vi "Begin.vi"(8 "error in":errorcluster) -> (0 "error out":errorcluster)   [LabVIEW 2018]
doc: "Called before other user functions, this VI is expected to open initial I/O refnums, load in file data, and do all program initialization. Notice that the <B>error out</B> terminal is simply used for data flow. Wiring it to other structures or subVIs ensures that this VI runs first."
uses:
  <vilib>/Rock Robotics/WPI/SafetyOutput/WPI_SafetyOutputConfigMenu.ctl
  <vilib>/Rock Robotics/WPI/DriverStation/WPI_DriverStationRobotMode2.ctl
  <vilib>/Rock Robotics/WPI/Joystick/WPI_JoystickDeviceEnum.ctl
  <vilib>/Rock Robotics/SystemInterfaces/DIO/FPGA_DIOPWMChannel.ctl
  Robot Global Data.vi
  <vilib>/Rock Robotics/Network Tables/NT Write String Array.vi
  <vilib>/Rock Robotics/WPI/RobotDrive/WPI_RobotDriveOpen4MotorWithJaguar.vi
  <vilib>/Rock Robotics/WPI/Solenoid/WPI_SolenoidChannel.ctl
  <vilib>/Rock Robotics/WPI/MotorControl/WPI_MotorControlOpen SPARK.vi
  <vilib>/Rock Robotics/WPI/Solenoid/WPI_SolenoidOpenDouble.vi
  <vilib>/Rock Robotics/WPI/ThirdParty/REV Robotics/SPARK MAX/Typedef/Spark MAX Motor Type.ctl
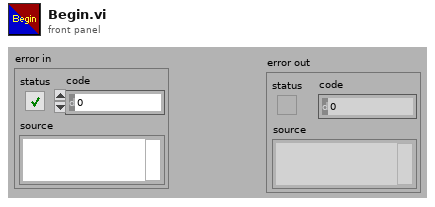
[diagram p1: front panel]
types:
  T1 = typedef "FPGA_DIOPWMChannel.ctl" = enum8{"PWM 0", "PWM 1", "PWM 2", "PWM 3", "PWM 4", "PWM 5", "PWM 6", "PWM 7", "PWM 8", "PWM 9", "PWM MXP 0", "PWM MXP 1", "PWM MXP 2", "PWM MXP 3", "PWM MXP 4", "PWM MXP 5", "PWM MXP 6", "PWM MXP 7", "PWM MXP 8", "PWM MXP 9", "Invalid"}
  T2 = typedef "WPI_JoystickDeviceEnum.ctl" = enum16{"USB 0", "USB 1", "USB 2", "USB 3", "USB 4", "USB 5"}
  T3 = typedef "WPI_DriverStationRobotMode2.ctl" = enum16{"Autonomous Disabled", "Autonomous Enabled", "Teleop Disabled", "Teleop Enabled", "Disconnected", "Finish", "Test Disabled", "Test Enabled", "Emergency Stopped"}
  T4 = typedef "WPI_SafetyOutputConfigMenu.ctl" = enum16{"Enable", "Disable"}
  T5 = typedef "Spark MAX Motor Type.ctl" = enum16{"Brushed", "Brushless"}
  T6 = cluster{"P Gain":dbl, "I Gain":dbl, "D Gain":dbl, "F Gain":dbl, "I Zone":dbl, "Min Output":dbl, "Max Output":dbl}
  T7 = typedef "WPI_SolenoidChannel.ctl" = enum8{"Solenoid 0", "Solenoid 1", "Solenoid 2", "Solenoid 3", "Solenoid 4", "Solenoid 5", "Solenoid 6", "Solenoid 7", "Invalid"}
  T8 = typedef "WPI_MotorControlDeviceRef.ctl" = cluster{"DeviceStatus":errorcluster, "Type":T9, "PWM":cluster{"PWM Channel":T1, "DeadBand":T10}, "CAN":cluster{"Device Number":u8, "SetOutput VI Ref":variant, "GetOutput VI Ref":variant, "Enable VI Ref":variant, "Disable VI Ref":variant, "Data":variant}, "Invert":bool, "DIO PWM":cluster{"PWM \"Enable\" Channel":T1, "DIOChannel":T11, "PWM Rate":dbl}}
  T9 = typedef "WPI_MotorControlType.ctl" = enum16{"PWM", "CAN", "DIO PWM"}
  T10 = typedef "WPI_PWMDeadband.ctl" = cluster{"Name":string, "maxPositivePwm":i32, "minPositivePwm":i32, "centerPwm":i32, "maxNegativePwm":i32, "minNegativePwm":i32, "angularRange":u16}
  T11 = typedef "FPGA_DIOChannel.ctl" = enum8{"DIO 0", "DIO 1", "DIO 2", "DIO 3", "DIO 4", "DIO 5", "DIO 6", "DIO 7", "DIO 8", "DIO 9", "DIO MXP 0", "DIO MXP 1", "DIO MXP 2", "DIO MXP 3", "DIO MXP 4", "DIO MXP 5", "DIO MXP 6", "DIO MXP 7", "DIO MXP 8", "DIO MXP 9", "DIO MXP 10", "DIO MXP 11", "DIO MXP 12", "DIO MXP 13", "DIO MXP 14", "DIO MXP 15", "SPI Port CS1", "SPI Port CS2", "SPI Port CS3", "SPI Port MISO", "SPI Port MOSI", "Invalid"}
  T12 = typedef "WPI_SolenoidDevRef.ctl" = cluster{"DevStatus":errorcluster, "Pneumatics Control Module":u8, "Forward Solenoid Channel":T7, "Reverse Solenoid Channel":T7}
  T13 = typedef "WPI_CompressorDevRef.ctl" = cluster{"DevStatus":errorcluster, "Pneumatics Control Module":u8}
  T14 = typedef "WPI_CameraDevRef.ctl" = cluster{"Camera Address":string, "CameraStatus":errorcluster}
  T15 = typedef "WPI_RobotDriveDevRef.ctl" = cluster{"DevStatus":errorcluster, "Motors[]":T8[], "Square Inputs":bool, "Max Output":dbl}
  T16 = typedef "WPI_JoystickDevRef.ctl" = cluster{"Device":T2}
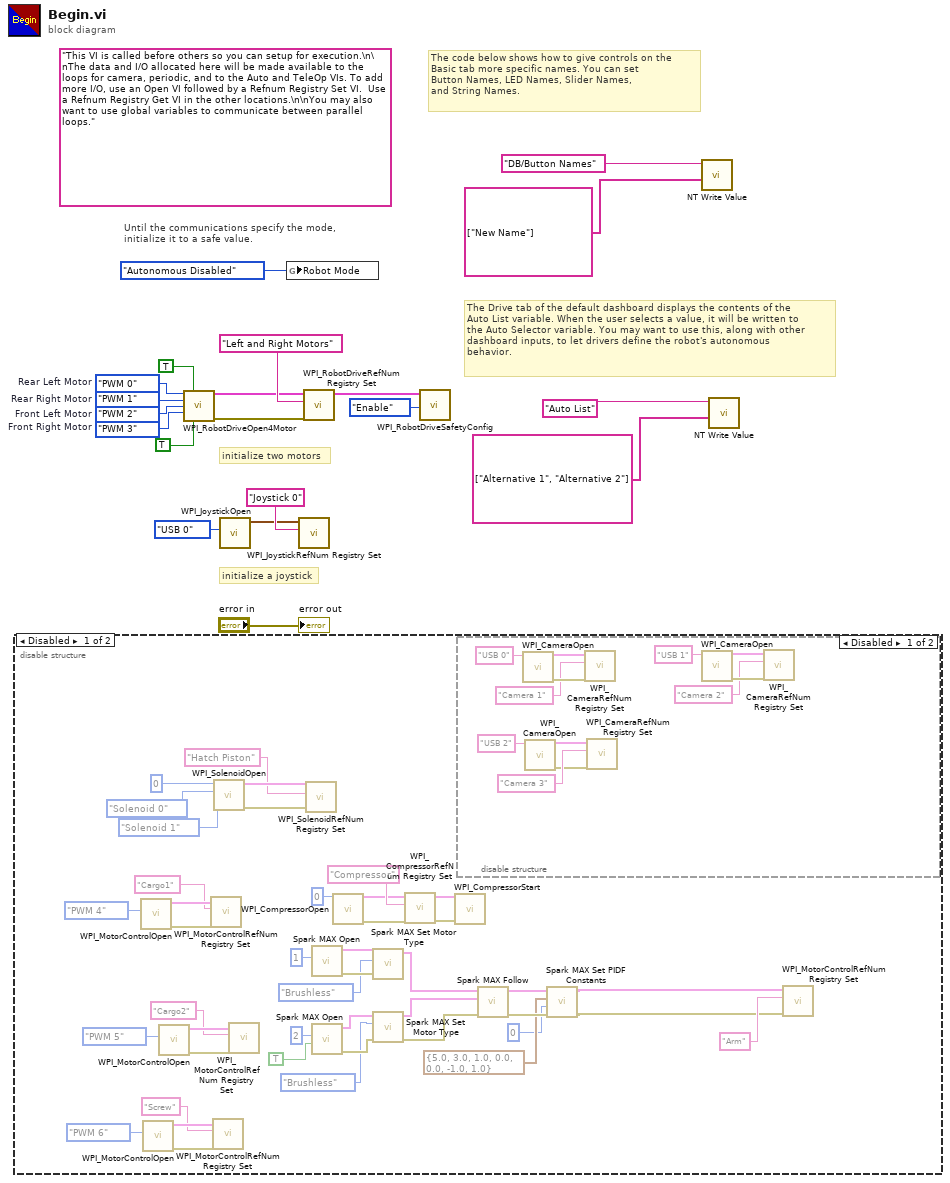
[diagram p0: block diagram]
diagram:
  w3 = FPGA_DIOPWMChannel."PWM 3"  # Front Right Motor
  w4 = FPGA_DIOPWMChannel."PWM 2"  # Front Left Motor
  w5 = FPGA_DIOPWMChannel."PWM 1"  # Rear Right Motor
  w6 = FPGA_DIOPWMChannel."PWM 0"  # Rear Left Motor
  (unwired) "This VI is called before others so you can setup for execution.\n\nThe data and I/O allocated here will be made available to the loops for camera, periodic, and to the Auto and TeleOp VIs. To add more I/O, use an Open VI followed by a Refnum Registry Set VI.  Use a Refnum Registry Get VI in the other locations.\n\nYou may also want to use global variables to communicate between parallel loops."
  # "The Drive tab of the default dashboard displays the contents of the\nAuto List variable. When the user selects a value, it will be written to\nthe Auto Selector variable. You may want to use this, along with other\ndashboard inputs, to let drivers define the robot's autonomous\nbehavior."
  # "The code below shows how to give controls on the\nBasic tab more specific names. You can set\nButton Names, LED Names, Slider Names,\nand String Names."
  # "initialize a joystick"
  # "Until the communications specify the mode,\ninitialize it to a safe value."
  # "initialize two motors"
  n1 = disable-structure shown="Disabled" {
    frame Disabled {
      n2 = call-poly <vilib>:"WPI_MotorControlOpen.vi"("PWM Channel"=FPGA_DIOPWMChannel."PWM 4") -> ("error out"=w58:errorcluster, "MotorControlDeviceRef"=w57:T8)  [unwired: 9 in]
      n3 = call-poly <vilib>:"WPI_MotorControlOpen.vi"("PWM Channel"=FPGA_DIOPWMChannel."PWM 6") -> ("error out"=w24:errorcluster, "MotorControlDeviceRef"=w23:T8)  [unwired: 9 in]
      n4 = call-poly <vilib>:"WPI_MotorControlOpen.vi"("PWM Channel"=FPGA_DIOPWMChannel."PWM 5") -> ("error out"=w47:errorcluster, "MotorControlDeviceRef"=w46:T8)  [unwired: 9 in]
      n5 = call <vilib>:"WPI_MotorControlRefNum Registry Set.vi"("error in (no error)"=w58, "refnum name"="Cargo1", "MotorControlDevRef"=w57) -> ()  [unwired: 7 in, 2 out]
      n6 = call <vilib>:"WPI_MotorControlRefNum Registry Set.vi"("error in (no error)"=w24, "refnum name"="Screw", "MotorControlDevRef"=w23) -> ()  [unwired: 7 in, 2 out]
      n7 = call-poly <vilib>:"WPI_SolenoidOpen.vi"("Reverse Solenoid Channel"=WPI_SolenoidChannel."Solenoid 1", "Forward Solenoid Channel"=WPI_SolenoidChannel."Solenoid 0" ("Solenoid Channel"), "Pneumatics Control Module (0)"=u8 0) -> ("error out"=w60:errorcluster, "SolenoidDevRef"=w63:T12)  [unwired: 7 in]
      n8 = call <vilib>:"WPI_MotorControlRefNum Registry Set.vi"("error in (no error)"=w47, "refnum name"="Cargo2", "MotorControlDevRef"=w46) -> ()  [unwired: 7 in, 2 out]
      n9 = call <vilib>:"WPI_SolenoidRefNum Registry Set.vi"("error in (no error)"=w60, "refnum name"="Hatch Piston", "SolenoidDevRef"=w63) -> ()  [unwired: 7 in, 2 out]
      n10 = call <vilib>:"Spark MAX Open.vi"("Device Number"=u8 1) -> ("error out"=w34:errorcluster, "MotorControlDeviceRef"=w35:T8)  [unwired: 9 in]
      n11 = call <vilib>:"Spark MAX Open.vi"("Invert"=TRUE, "Device Number"=u8 2) -> ("error out"=w28:errorcluster, "MotorControlDeviceRef"=w29:T8)  [unwired: 8 in]
      n12 = call <vilib>:"WPI_CompressorOpen.vi"("Pneumatics Control Module (0)"=u8 0) -> ("CompressorDevRef"=w51:T13, "error out"=w54:errorcluster)  [unwired: 13 in]
      n13 = call <vilib>:"Spark MAX Set Motor Type.vi"("error in (no error)"=w34, "Enum"=Spark_MAX_Motor_Type."Brushless", "MotorControlDevRef"=w35) -> ("MotorControlDeviceRef"=w32:T8)  [unwired: 7 in, 1 out]
      n14 = call <vilib>:"Spark MAX Set Motor Type.vi"("error in (no error)"=w28, "Enum"=Spark_MAX_Motor_Type."Brushless", "MotorControlDevRef"=w29) -> ("error out"=w30:errorcluster, "MotorControlDeviceRef"=w31:T8)  [unwired: 7 in]
      n15 = call <vilib>:"WPI_CompressorRefNum Registry Set.vi"("error in (no error)"=w54, "refnum name"="Compressor", "CompressorDevRef"=w51) -> ("error out"=w50:errorcluster, "CompressorDevRef"=w49:T13)  [unwired: 7 in]
      n16 = call <vilib>:"WPI_CompressorStart.vi"("error in (no error)"=w50, "CompressorDevRef"=w49) -> ()  [unwired: 8 in, 2 out]
      n17 = disable-structure shown="Disabled" {
        frame Disabled {
          n18 = call <vilib>:"WPI_CameraOpen.vi"("Camera Address"="USB 0") -> ("error out"=w73:errorcluster, "CameraDevRef"=w74:T14)  [unwired: 9 in]
          n19 = call <vilib>:"WPI_CameraOpen.vi"("Camera Address"="USB 2") -> ("error out"=w70:errorcluster, "CameraDevRef"=w69:T14)  [unwired: 9 in]
          n20 = call <vilib>:"WPI_CameraRefNum Registry Set.vi"("error in (no error)"=w73, "refnum name"="Camera 1", "CameraDevRef"=w74) -> ()  [unwired: 7 in, 2 out]
          n21 = call <vilib>:"WPI_CameraRefNum Registry Set.vi"("error in (no error)"=w70, "refnum name"="Camera 3", "CameraDevRef"=w69) -> ()  [unwired: 7 in, 2 out]
          n22 = call <vilib>:"WPI_CameraOpen.vi"("Camera Address"="USB 1") -> ("error out"=w65:errorcluster, "CameraDevRef"=w66:T14)  [unwired: 9 in]
          n23 = call <vilib>:"WPI_CameraRefNum Registry Set.vi"("error in (no error)"=w65, "refnum name"="Camera 2", "CameraDevRef"=w66) -> ()  [unwired: 7 in, 2 out]
        }
        frame Enabled {
        }
      }
      n24 = call <vilib>:"Spark MAX Follow.vi"("error in (no error)"=w30, "Master Controller"=w31, "MotorControlDeviceRef"=w32) -> ("error out"=w38:errorcluster, "MotorControlDeviceRef"=w39:T8)  [unwired: 7 in]
      n25 = call <vilib>:"Spark MAX Set PIDF Constants.vi"("error in"=w38, "PIDF Slot"=0, "PID Constants"=T6 {"P Gain"=5.0, "I Gain"=3.0, "D Gain"=1.0, "F Gain"=0.0, "I Zone"=0.0, "Min Output"=-1.0, "Max Output"=1.0}, "MotorControlDeviceRef"=w39) -> ("error out"=w25:errorcluster, "MotorControlDeviceRef"=w26:T8)  [unwired: 6 in]
      n26 = call <vilib>:"WPI_MotorControlRefNum Registry Set.vi"("error in (no error)"=w25, "refnum name"="Arm", "MotorControlDevRef"=w26) -> ()  [unwired: 7 in, 2 out]
    }
    frame Enabled {
    }
  }
  n27 = call-poly <vilib>:"WPI_RobotDriveOpen4Motor.vi"("Rear Left Motor"=w6, "Rear Left Motor Inverted"=TRUE, "Rear Right Motor"=w5, "Front Left Motor"=w4, "Front Right Motor"=w3, "Front Left Motor Inverted"=TRUE) -> ("RobotDriveDevRef"=w8:T15, "error out"=w7:errorcluster)  [unwired: 8 in]
  n28 = call <vilib>:"WPI_JoystickOpen.vi"("JoystickDevice"=WPI_JoystickDeviceEnum."USB 0") -> ("JoystickDevRef"=w15:T16)  [unwired: 10 in]
  n29 = global write "Robot Global Data.vi" "Robot Mode"(WPI_DriverStationRobotMode2."Autonomous Disabled" ("Robot Mode")) -> ()
  n30 = call <vilib>:"WPI_JoystickRefNum Registry Set.vi"("refnum name"="Joystick 0", "JoystickDevRef"=w15) -> ()  [unwired: 8 in, 2 out]
  n31 = call <vilib>:"WPI_RobotDriveRefNum Registry Set.vi"("error in (no error)"=w7, "refnum name"="Left and Right Motors", "RobotDriveDevRef"=w8) -> ("RobotDriveDevRef"=w19:T15)  [unwired: 1 in, 7 out]
  n32 = call <vilib>:"WPI_RobotDriveSafetyConfig.vi"("mode"=WPI_SafetyOutputConfigMenu."Enable", "RobotDriveDevRef"=w19) -> ()  [unwired: 8 in, 2 out]
  n33 = call-poly <vilib>:"NT Write Value.vi"("String Array"=string[] ["New Name"], "Name"="DB/Button Names") -> ()  [unwired: 9 in, 1 out]
  n34 = call-poly <vilib>:"NT Write Value.vi"("String Array"=string[] ["Alternative 1", "Alternative 2"], "Name"="Auto List") -> ()  [unwired: 9 in, 1 out]
  "error out" <- "error in"
